vi "test_read-nmea-data2.vi"() -> ()   [LabVIEW 2019] (continued)
A,3,12,06,19,05,17,09,04,02,,,,,1.88,0.95,1.62,1*08\n\t\n15:13:30.30\tF9P\t$GNGSA,A,3,85,70,71,84,,,,,,,,,1.88,0.95,1.62,2*0A\n\t\n15:13:30.32\tF9P\t$GNGSA,A,3,36,19,11,04,09,12,,,,,,,1.88,0.95,1.62,3*08\n\t\n15:13:30.34\tF9P\t$GNGSA,A,3,14,11,33,,,,,,,,,,1.88,0.95,1.62,4*09\n\t\n15:13:30.36\tF9P\t$GPGSV,3,1,09,02,55,320,27,04,17,043,22,05,38,248,31,06,64,050,28,1*65\n\t\n15:13:30.38\tF9P\t$GPGSV,3,2,09,09,44,073,34,12,23,276,36,17,33,154,44,19,52,157,39,1*62\n\t\n15:13:30.40\tF9P\t$GPGSV,3,3,09,25,12,306,24,1*5A\n\t\n15:13:30.42\tF9P\t$GPGSV,3,1,09,02,55,320,,04,17,043,15,05,38,248,15,06,64,050,24,6*69\n\t\n15:13:30.44\tF9P\t$GPGSV,3,2,09,09,44,073,26,12,23,276,22,17,33,154,26,19,52,157,,6*6D\n\t\n15:13:30.46\tF9P\t$GPGSV,3,3,09,25,12,306,,6*5B\n\t\n15:13:30.48\tF9P\t$GLGSV,2,1,08,69,11,031,28,70,70,038,23,71,53,206,28,72,05,210,19,1*7B\n\t\n15:13:30.50\tF9P\t$GLGSV,2,2,08,77,01,325,,84,19,123,21,85,70,070,32,86,37,330,,1*74\n\t\n15:13:30.52\tF9P\t$GLGSV,2,1,08,69,11,031,30,70,70,038,,71,53,206,20,72,05,210,,3*71\n\t\n15:13:30.54\tF9P\t$GLGSV,2,2,08,77,01,325,,84,19,123,27,85,70,070,23,86,37,330,,3*70\n\t\n15:13:30.56\tF9P\t$GAGSV,2,1,08,02,08,297,09,04,66,116,27,09,32,193,27,11,72,359,23,7*7D\n\t\n15:13:30.58\tF9P\t$GAGSV,2,2,08,12,40,103,33,19,26,045,15,25,09,249,17,36,26,308,16,7*7D\n\t\n15:13:30.60\tF9P\t$GAGSV,2,1,08,02,08,297,,04,66,116,,09,32,193,,11,72,359,,2*70\n\t\n15:13:30.62\tF9P\t$GAGSV,2,2,08,12,40,103,,19,26,045,,25,09,249,,36,26,308,,2*7D\n\t\n15:13:30.64\tF9P\t$GBGSV,1,1,04,11,49,132,33,14,87,114,26,28,,,28,33,61,220,27,1*47\n\t\n15:13:30.66\tF9P\t$GBGSV,1,1,03,11,49,132,31,14,87,114,23,33,61,220,,3*40\n\t\n15:13:30.68\tF9P\t$GNGLL,3723.56358,N,12656.98749,E,061332.00,A,A*77\n\t\n15:13:30.70\tF9P\t\t\n15:13:30.72\tF9P\t\t\n15:13:30.74\tF9P\t\t\n15:13:30.76\tF9P\t\t\n15:13:30.78\tF9P\t\t\n15:13:30.80\tF9P\t\t\n15:13:30.82\tF9P\t\t\n15:13:30.84\tF9P\t\t\n15:13:30.86\tF9P\t\t\n15:13:30.88\tF9P\t\t\n15:13:30.90\tF9P\t\t\n15:13:30.92\tF9P\t\t\n15:13:30.94\tF9P\t\t\n15:13:30.96\tF9P\t\t\n15:13:30.98\tF9P\t\t\n15:13:31.00\tF9P\t\t\n15:13:31.02\tF9P\t\t\n15:13:31.04\tF9P\t\t\n15:13:31.06\tF9P\t\t\n15:13:31.08\tF9P\t\t\n15:13:31.10\tF9P\t\t\n15:13:31.12\tF9P\t\t\n15:13:31.14\tF9P\t\t\n15:13:31.16\tF9P\t\t\n15:13:31.18\tF9P\t\t\n15:13:31.20\tF9P\t\t\n15:13:31.22\tF9P\t\t\n15:13:31.24\tF9P\t$GNRMC,061333.00,A,3723.56413,N,12656.98779,E,2.031,10.66,250720,,,A,V*33\n\t\n15:13:31.26\tF9P\t$GNVTG,10.66,T,,M,2.031,N,3.761,K,A*11\n\t\n15:13:31.28\tF9P\t$GNGGA,061333.00,3723.56413,N,12656.98779,E,1,12,0.82,49.3,M,18.5,M,,*73\n\t\n15:13:31.30\tF9P\t$GNGSA,A,3,12,06,19,05,17,09,04,02,,,,,1.52,0.82,1.28,1*07\n\t\n15:13:31.32\tF9P\t$GNGSA,A,3,85,70,71,84,,,,,,,,,1.52,0.82,1.28,2*05\n\t\n15:13:31.34\tF9P\t$GNGSA,A,3,36,19,11,04,09,12,,,,,,,1.52,0.82,1.28,3*07\n\t\n15:13:31.36\tF9P\t$GNGSA,A,3,14,11,33,,,,,,,,,,1.52,0.82,1.28,4*06\n\t\n15:13:31.38\tF9P\t$GPGSV,3,1,09,02,55,320,26,04,17,043,22,05,38,248,25,06,64,050,28,1*61\n\t\n15:13:31.40\tF9P\t$GPGSV,3,2,09,09,44,073,26,12,23,276,33,17,33,154,42,19,52,157,31,1*6A\n\t\n15:13:31.42\tF9P\t$GPGSV,3,3,09,25,12,306,31,1*5E\n\t\n15:13:31.44\tF9P\t$GPGSV,3,1,09,02,55,320,,04,17,043,14,05,38,248,10,06,64,050,24,6*6D\n\t\n15:13:31.46\tF9P\t$GPGSV,3,2,09,09,44,073,26,12,23,276,20,17,33,154,25,19,52,157,,6*6C\n\t\n15:13:31.48\tF9P\t$GPGSV,3,3,09,25,12,306,,6*5B\n\t\n15:13:31.50\tF9P\t$GLGSV,2,1,08,69,11,031,25,70,70,038,22,71,53,206,27,72,05,210,18,1*79\n\t\n15:13:31.52\tF9P\t$GLGSV,2,2,08,77,01,325,,84,19,123,21,85,70,070,32,86,37,330,,1*74\n\t\n15:13:31.54\tF9P\t$GLGSV,2,1,08,69,11,031,26,70,70,038,,71,53,206,19,72,05,210,,3*7C\n\t\n15:13:31.56\tF9P\t$GLGSV,2,2,08,77,01,325,,84,19,123,26,85,70,070,21,86,37,330,,3*73\n\t\n15:13:31.58\tF9P\t$GAGSV,2,1,08,02,08,297,07,04,66,116,27,09,32,193,27,11,72,359,24,7*74\n\t\n15:13:31.60\tF9P\t$GAGSV,2,2,08,12,40,103,29,19,26,045,15,25,09,249,13,36,26,308,16,7*72\n\t\n15:13:31.62\tF9P\t$GAGSV,2,1,08,02,08,297,,04,66,116,,09,32,193,,11,72,359,,2*70\n\t\n15:13:31.64\tF9P\t$GAGSV,2,2,08,12,40,103,,19,26,045,,25,09,249,,36,26,308,,2*7D\n\t\n15:13:31.66\tF9P\t$GBGSV,1,1,04,11,49,132,36,14,87,114,27,28,,,27,33,61,220,27,1*4C\n\t\n15:13:31.68\tF9P\t$GBGSV,1,1,03,11,49,132,30,14,87,114,30,33,61,220,,3*43\n\t\n15:13:31.70\tF9P\t$GNGLL,3723.56413,N,12656.98779,E,061333.00,A,A*7D\n\t\n15:13:31.72\tF9P\t\t\n15:13:31.74\tF9P\t\t\n15:13:31.76\tF9P\t\t\n15:13:31.78\tF9P\t\t\n15:13:31.80\tF9P\t\t\n15:13:31.82\tF9P\t\t\n15:13:31.84\tF9P\t\t\n15:13:31.86\tF9P\t\t\n15:13:31.88\tF9P\t\t\n15:13:31.90\tF9P\t\t\n15:13:31.92\tF9P\t\t\n15:13:31.94\tF9P\t\t\n15:13:31.96\tF9P\t\t\n15:13:31.98\tF9P\t\t\n15:13:32.00\tF9P\t\t\n15:13:32.02\tF9P\t\t\n15:13:32.04\tF9P\t\t\n15:13:32.06\tF9P\t\t\n15:13:32.08\tF9P\t\t\n15:13:32.10\tF9P\t\t\n15:13:32.12\tF9P\t\t\n15:13:32.14\tF9P\t\t\n15:13:32.16\tF9P\t\t\n15:13:32.18\tF9P\t\t\n15:13:32.20\tF9P\t\t\n15:13:32.22\tF9P\t\t\n15:13:32.24\tF9P\t$GNRMC,061334.00,A,3723.56475,N,12656.98800,E,1.899,7.08,250720,,,A,V*02\n\t\n15:13:32.26\tF9P\t$GNVTG,7.08,T,,M,1.899,N,3.517,K,A*25\n\t\n15:13:32.28\tF9P\t$GNGGA,061334.00,3723.56475,N,12656.98800,E,1,12,0.82,49.2,M,18.5,M,,*74\n\t\n15:13:32.30\tF9P\t$GNGSA,A,3,12,06,19,05,17,09,04,02,,,,,1.52,0.82,1.28,1*07\n\t\n15:13:32.32\tF9P\t$GNGSA,A,3,85,70,71,84,,,,,,,,,1.52,0.82,1.28,2*05\n\t\n15:13:32.34\tF9P\t$GNGSA,A,3,36,19,11,04,09,12,,,,,,,1.52,0.82,1.28,3*07\n\t\n15:13:32.36\tF9P\t$GNGSA,A,3,14,11,33,,,,,,,,,,1.52,0.82,1.28,4*06\n\t\n15:13:32.38\tF9P\t$GPGSV,3,1,09,02,55,320,31,04,17,043,22,05,38,248,24,06,64,050,33,1*6C\n\t\n15:13:32.40\tF9P\t$GPGSV,3,2,09,09,44,073,31,12,23,276,37,17,32,154,31,19,52,157,35,1*69\n\t\n15:13:32.42\tF9P\t$GPGSV,3,3,09,25,12,306,24,1*5A\n\t\n15:13:32.44\tF9P\t$GPGSV,3,1,09,02,55,320,,04,17,043,12,05,38,248,,06,64,050,24,6*6A\n\t\n15:13:32.46\tF9P\t$GPGSV,3,2,09,09,44,073,26,12,23,276,20,17,32,154,25,19,52,157,,6*6D\n\t\n15:13:32.48\tF9P\t$GPGSV,3,3,09,25,12,306,,6*5B\n\t\n15:13:32.50\tF9P\t$GLGSV,2,1,08,69,11,031,31,70,70,038,22,71,53,206,28,72,05,210,17,1*7C\n\t\n15:13:32.52\tF9P\t$GLGSV,2,2,08,77,01,325,,84,19,123,19,85,70,070,33,86,37,330,,1*7E\n\t\n15:13:32.54\tF9P\t$GLGSV,2,1,08,69,11,031,26,70,70,038,,71,53,206,18,72,05,210,,3*7D\n\t\n15:13:32.56\tF9P\t$GLGSV,2,2,08,77,01,325,,84,19,123,25,85,70,070,21,86,37,330,,3*70\n\t\n15:13:32.58\tF9P\t$GAGSV,2,1,08,02,08,297,08,04,66,116,31,09,32,193,25,11,72,359,24,7*7E\n\t\n15:13:32.60\tF9P\t$GAGSV,2,2,08,12,40,103,29,19,26,045,16,25,09,249,11,36,26,308,15,7*70\n\t\n15:13:32.62\tF9P\t$GAGSV,2,1,08,02,08,297,,04,66,116,,09,32,193,,11,72,359,,2*70\n\t\n15:13:32.64\tF9P\t$GAGSV,2,2,08,12,40,103,,19,26,045,,25,09,249,,36,26,308,,2*7D\n\t\n15:13:32.66\tF9P\t$GBGSV,1,1,04,11,49,132,33,14,87,114,28,28,,,26,33,61,220,38,1*49\n\t\n15:13:32.68\tF9P\t$GBGSV,1,1,03,11,49,132,,14,87,114,,33,61,220,,3*43\n\t\n15:13:32.70\tF9P\t$GNGLL,3723.56475,N,12656.98800,E,061334.00,A,A*7B\n\t\n15:13:32.72\tF9P\t\t\n15:13:32.74\tF9P\t\t\n15:13:32.76\tF9P\t\t\n15:13:32.78\tF9P\t\t\n15:13:32.80\tF9P\t\t\n15:13:32.82\tF9P\t\t\n15:13:32.84\tF9P\t\t\n15:13:32.86\tF9P\t\t\n15:13:32.88\tF9P\t\t\n15:13:32.90\tF9P\t\t\n15:13:32.92\tF9P\t\t\n15:13:32.94\tF9P\t\t\n15:13:32.96\tF9P\t\t\n15:13:32.98\tF9P\t\t\n15:13:33.00\tF9P\t\t\n15:13:33.02\tF9P\t\t\n15:13:33.04\tF9P\t\t\n15:13:33.06\tF9P\t\t\n15:13:33.08\tF9P\t\t\n15:13:33.10\tF9P\t\t\n15:13:33.12\tF9P\t\t\n15:13:33.14\tF9P\t\t\n15:13:33.16\tF9P\t\t\n15:13:33.18\tF9P\t\t\n15:13:33.20\tF9P\t\t\n15:13:33.22\tF9P\t\t\n15:13:33.24\tF9P\t$GNRMC,061335.00,A,3723.56544,N,12656.98826,E,2.231,5.91,250720,,,A,V*0D\n\t\n15:13:33.26\tF9P\t$GNVTG,5.91,T,,M,2.231,N,4.131,K,A*2B\n\t\n15:13:33.28\tF9P\t$GNGGA,061335.00,3723.56544,N,12656.98826,E,1,12,0.95,49.1,M,18.5,M,,*77\n\t\n15:13:33.30\tF9P\t$GNGSA,A,3,12,06,19,05,17,09,04,02,,,,,1.88,0.95,1.62,1*08\n\t\n15:13:33.32\tF9P\t$GNGSA,A,3,85,70,71,84,,,,,,,,,1.88,0.95,1.62,2*0A\n\t\n15:13:33.34\tF9P\t$GNGSA,A,3,36,19,11,04,09,12,,,,,,,1.88,0.95,1.62,3*08\n\t\n15:13:33.36\tF9P\t$GNGSA,A,3,14,11,33,,,,,,,,,,1.88,0.95,1.62,4*09\n\t\n15:13:33.38\tF9P\t$GPGSV,3,1,09,02,55,320,32,04,17,043,22,05,38,248,25,06,64,050,33,1*6E\n\t\n15:13:33.40\tF9P\t$GPGSV,3,2,09,09,44,073,30,12,23,276,35,17,32,154,39,19,52,157,33,1*64\n\t\n15:13:33.42\tF9P\t$GPGSV,3,3,09,25,12,306,22,1*5C\n\t\n15:13:33.44\tF9P\t$GPGSV,3,1,09,02,55,320,,04,17,043,10,05,38,248,,06,64,050,31,6*6C\n\t\n15:13:33.46\tF9P\t$GPGSV,3,2,09,09,44,073,25,12,23,276,19,17,32,154,25,19,52,157,,6*64\n\t\n15:13:33.48\tF9P\t$GPGSV,3,3,09,25,12,306,,6*5B\n\t\n15:13:33.50\tF9P\t$GLGSV,2,1,08,69,11,031,29,70,70,038,23,71,53,206,35,72,05,210,17,1*78\n\t\n15:13:33.52\tF9P\t$GLGSV,2,2,08,77,01,325,,84,19,123,18,85,70,070,35,86,37,330,,1*79\n\t\n15:13:33.54\tF9P\t$GLGSV,2,1,08,69,11,031,25,70,70,038,,71,53,206,21,72,05,210,,3*74\n\t\n15:13:33.56\tF9P\t$GLGSV,2,2,08,77,01,325,,84,19,123,22,85,70,070,21,86,37,330,,3*77\n\t\n15:13:33.58\tF9P\t$GAGSV,2,1,08,02,08,297,11,04,66,116,24,09,32,193,25,11,72,359,25,7*73\n\t\n15:13:33.60\tF9P\t$GAGSV,2,2,08,12,40,103,28,19,26,045,16,25,09,249,10,36,26,308,14,7*71\n\t\n15:13:33.62\tF9P\t$GAGSV,2,1,08,02,08,297,,04,66,116,,09,32,193,,11,72,359,,2*70\n\t\n15:13:33.64\tF9P\t$GAGSV,2,2,08,12,40,103,,19,26,045,,25,09,249,,36,26,308,,2*7D\n\t\n15:13:33.66\tF9P\t$GBGSV,1,1,04,11,49,132,38,14,87,114,27,28,,,26,33,61,220,35,1*40\n\t\n15:13:33.68\tF9P\t$GBGSV,1,1,03,11,49,132,29,14,87,114,,33,61,220,,3*48\n\t\n15:13:33.70\tF9P\t$GNGLL,3723.56544,N,12656.98826,E,061335.00,A,A*7D\n\t\n15:13:33.72\tF9P\t\t\n15:13:33.74\tF9P\t\t\n15:13:33.76\tF9P\t\t\n15:13:33.78\tF9P\t\t\n15:13:33.80\tF9P\t\t\n15:13:33.82\tF9P\t\t\n15:13:33.84\tF9P\t\t\n15:13:33.86\tF9P\t\t\n15:13:33.88\tF9P\t\t\n15:13:33.90\tF9P\t\t\n15:13:33.92\tF9P\t\t\n15:13:33.94\tF9P\t\t\n15:13:33.96\tF9P\t\t\n15:13:33.98\tF9P\t\t\n15:13:34.00\tF9P\t\t\n15:13:34.02\tF9P\t\t\n15:13:34.04\tF9P\t\t\n15:13:34.06\tF9P\t\t\n15:13:34.08\tF9P\t\t\n15:13:34.10\tF9P\t\t\n15:13:34.12\tF9P\t\t\n15:13:34.14\tF9P\t\t\n15:13:34.16\tF9P\t\t\n15:13:34.18\tF9P\t\t\n15:13:34.20\tF9P\t\t\n15:13:34.22\tF9P\t\t\n15:13:34.24\tF9P\t$GNRMC,061336.00,A,3723.56612,N,12656.98828,E,1.880,2.24,250720,,,A,V*0A\n\t\n15:13:34.26\tF9P\t$GNVTG,2.24,T,,M,1.880,N,3.482,K,A*2B\n\t\n15:13:34.28\tF9P\t$GNGGA,061336.00,3723.56612,N,12656.98828,E,1,12,1.09,48.9,M,18.5,M,,*77\n\t\n15:13:34.30\tF9P\t$GNGSA,A,3,12,06,19,05,17,09,04,02,,,,,2.14,1.09,1.84,1*02\n\t\n15:13:34.32\tF9P\t$GNGSA,A,3,85,70,71,84,,,,,,,,,2.14,1.09,1.84,2*00\n\t\n15:13:34.35\tF9P\t$GNGSA,A,3,36,19,11,04,09,12,,,,,,,2.14,1.09,1.84,3*02\n\t\n15:13:34.37\tF9P\t$GNGSA,A,3,14,11,33,,,,,,,,,,2.14,1.09,1.84,4*03\n\t\n15:13:34.39\tF9P\t$GPGSV,3,1,09,02,55,320,32,04,17,043,20,05,38,248,26,06,64,050,28,1*65\n\t\n15:13:34.41\tF9P\t$GPGSV,3,2,09,09,44,073,32,12,23,276,38,17,32,154,38,19,51,157,29,1*62\n\t\n15:13:34.43\tF9P\t$GPGSV,3,3,09,25,12,306,21,1*5F\n\t\n15:13:34.45\tF9P\t$GPGSV,3,1,09,02,55,320,,04,17,043,11,05,38,248,,06,64,050,25,6*68\n\t\n15:13:34.47\tF9P\t$GPGSV,3,2,09,09,44,073,25,12,23,276,19,17,32,154,24,19,51,157,,6*66\n\t\n15:13:34.49\tF9P\t$GPGSV,3,3,09,25,12,306,,6*5B\n\t\n15:13:34.51\tF9P\t$GLGSV,2,1,08,69,11,031,28,70,70,038,24,71,53,206,33,72,05,210,18,1*77\n\t\n15:13:34.53\tF9P\t$GLGSV,2,2,08,77,01,325,,84,19,123,19,85,70,070,38,86,37,330,,1*75\n\t\n15:13:34.55\tF9P\t$GLGSV,2,1,08,69,11,031,23,70,70,038,,71,53,206,25,72,05,210,,3*76\n\t\n15:13:34.57\tF9P\t$GLGSV,2,2,08,77,01,325,,84,19,123,21,85,70,070,21,86,37,330,,3*74\n\t\n15:13:34.59\tF9P\t$GAGSV,2,1,08,02,08,297,07,04,66,116,26,09,32,193,34,11,72,359,26,7*75\n\t\n15:13:34.61\tF9P\t$GAGSV,2,2,08,12,40,103,28,19,26,045,17,25,09,249,10,36,26,308,14,7*70\n\t\n15:13:34.63\tF9P\t$GAGSV,2,1,08,02,08,297,,04,66,116,,09,32,193,,11,72,359,,2*70\n\t\n15:13:34.65\tF9P\t$GAGSV,2,2,08,12,40,103,,19,26,045,,25,09,249,,36,26,308,,2*7D\n\t\n15:13:34.67\tF9P\t$GBGSV,1,1,04,11,49,132,30,14,87,114,27,28,,,27,33,61,220,33,1*4F\n\t\n15:13:34.69\tF9P\t$GBGSV,1,1,03,11,49,132,,14,87,114,,33,61,220,,3*43\n\t\n15:13:34.71\tF9P\t$GNGLL,3723.56612,N,12656.98828,E,061336.00,A,A*70\n\t\n15:13:34.73\tF9P\t\t\n15:13:34.75\tF9P\t\t\n15:13:34.77\tF9P\t\t\n15:13:34.79\tF9P\t\t\n15:13:34.81\tF9P\t\t\n15:13:34.83\tF9P\t\t\n15:13:34.85\tF9P\t\t\n15:13:34.87\tF9P\t\t\n15:13:34.89\tF9P\t\t\n15:13:34.91\tF9P\t\t\n15:13:34.93\tF9P\t\t\n15:13:34.95\tF9P\t\t\n15:13:34.97\tF9P\t\t\n15:13:34.99\tF9P\t\t\n15:13:35.01\tF9P\t\t\n15:13:35.03\tF9P\t\t\n15:13:35.05\tF9P\t\t\n15:13:35.07\tF9P\t\t\n15:13:35.09\tF9P\t\t\n15:13:35.11\tF9P\t\t\n15:13:35.13\tF9P\t\t\n15:13:35.15\tF9P\t\t\n15:13:35.17\tF9P\t\t\n15:13:35.19\tF9P\t\t\n15:13:35.21\tF9P\t\t\n15:13:35.23\tF9P\t$GNRMC,061337.00,A,3723.56656,N,12656.98836,E,1.514,358.52,250720,,,A,V*09\n\t\n15:13:35.25\tF9P\t$GNVTG,358.52,T,,M,1.514,N,2.804,K,A*25\n\t\n15:13:35.27\tF9P\t$GNGGA,061337.00,3723.56656,N,12656.98836,E,1,12,1.09,49.1,M,18.5,M,,*70\n\t\n15:13:35.29\tF9P\t$GNGSA,A,3,12,06,19,05,17,09,04,02,,,,,2.14,1.09,1.84,1*02\n\t\n15:13:35.31\tF9P\t$GNGSA,A,3,85,70,71,84,,,,,,,,,2.14,1.09,1.84,2*00\n\t\n15:13:35.33\tF9P\t$GNGSA,A,3,36,19,11,04,09,12,,,,,,,2.14,1.09,1.84,3*02\n\t\n15:13:35.35\tF9P\t$GNGSA,A,3,14,11,33,,,,,,,,,,2.14,1.09,1.84,4*03\n\t\n15:13:35.37\tF9P\t$GPGSV,3,1,09,02,55,320,27,04,17,043,19,05,38,248,26,06,64,050,34,1*66\n\t\n15:13:35.39\tF9P\t$GPGSV,3,2,09,09,44,073,27,12,23,276,31,17,32,154,31,19,51,157,32,1*6C\n\t\n15:13:35.41\tF9P\t$GPGSV,3,3,09,25,12,306,22,1*5C\n\t\n15:13:35.43\tF9P\t$GPGSV,3,1,09,02,55,320,,04,17,043,10,05,38,248,,06,64,050,26,6*6A\n\t\n15:13:35.45\tF9P\t$GPGSV,3,2,09,09,44,073,27,12,23,276,18,17,32,154,25,19,51,157,,6*64\n\t\n15:13:35.47\tF9P\t$GPGSV,3,3,09,25,12,306,,6*5B\n\t\n15:13:35.49\tF9P\t$GLGSV,2,1,08,69,11,031,28,70,70,038,25,71,53,206,31,72,05,210,18,1*74\n\t\n15:13:35.51\tF9P\t$GLGSV,2,2,08,77,01,325,,84,19,123,19,85,70,070,32,86,37,330,,1*7F\n\t\n15:13:35.53\tF9P\t$GLGSV,2,1,08,69,11,031,22,70,70,038,,71,53,206,25,72,05,210,,3*77\n\t\n15:13:35.55\tF9P\t$GLGSV,2,2,08,77,01,325,,84,19,123,21,85,70,070,24,86,37,330,,3*71\n\t\n15:13:35.57\tF9P\t$GAGSV,2,1,08,02,08,297,07,04,66,116,32,09,32,193,31,11,72,359,24,7*77\n\t\n15:13:35.59\tF9P\t$GAGSV,2,2,08,12,40,103,28,19,26,045,17,25,09,249,09,36,26,308,13,7*7F\n\t\n15:13:35.61\tF9P\t$GAGSV,2,1,08,02,08,297,,04,66,116,,09,32,193,,11,72,359,,2*70\n\t\n15:13:35.63\tF9P\t$GAGSV,2,2,08,12,40,103,,19,26,045,,25,09,249,,36,26,308,,2*7D\n\t\n15:13:35.65\tF9P\t$GBGSV,1,1,04,11,49,132,33,14,87,114,32,28,,,27,33,61,220,35,1*4E\n\t\n15:13:35.67\tF9P\t$GBGSV,1,1,03,11,49,132,,14,87,114,31,33,61,220,,3*41\n\t\n15:13:35.69\tF9P\t$GNGLL,3723.56656,N,12656.98836,E,061337.00,A,A*7E\n\t\n15:13:35.71\tF9P\t\t\n15:13:35.73\tF9P\t\t\n15:13:35.75\tF9P\t\t\n15:13:35.77\tF9P\t\t\n15:13:35.79\tF9P\t\t\n15:13:35.81\tF9P\t\t\n15:13:35.83\tF9P\t\t\n15:13:35.85\tF9P\t\t\n15:13:35.87\tF9P\t\t\n15:13:35.89\tF9P\t\t\n15:13:35.91\tF9P\t\t\n15:13:35.93\tF9P\t\t\n15:13:35.95\tF9P\t\t\n15:13:35.97\tF9P\t\t\n15:13:35.99\tF9P\t\t\n15:13:36.01\tF9P\t\t\n15:13:36.03\tF9P\t\t\n15:13:36.05\tF9P\t\t\n15:13:36.07\tF9P\t\t\n15:13:36.09\tF9P\t\t\n15:13:36.11\tF9P\t\t\n15:13:36.13\tF9P\t\t\n15:13:36.15\tF9P\t\t\n15:13:36.17\tF9P\t\t\n15:13:36.19\tF9P\t\t\n15:13:36.21\tF9P\t\t\n15:13:36.23\tF9P\t$GNRMC,061338.00,A,3723.56740,N,12656.98792,E,2.771,332.85,250720,,,A,V*05\n\t\n15:13:36.25\tF9P\t$GNVTG,332.85,T,,M,2.771,N,5.132,K,A*2A\n\t\n15:13:36.27\tF9P\t$GNGGA,061338.00,3723.56740,N,12656.98792,E,1,12,0.82,47.5,M,18.5,M,,*70\n\t\n15:13:36.29\tF9P\t$GNGSA,A,3,12,06,19,05,17,09,04,02,,,,,1.52,0.82,1.28,1*07\n\t\n15:13:36.31\tF9P\t$GNGSA,A,3,85,70,71,84,,,,,,,,,1.52,0.82,1.28,2*05\n\t\n15:13:36.33\tF9P\t$GNGSA,A,3,36,19,11,04,09,12,,,,,,,1.52,0.82,1.28,3*07\n\t\n15:13:36.35\tF9P\t$GNGSA,A,3,14,11,33,,,,,,,,,,1.52,0.82,1.28,4*06\n\t\n15:13:36.37\tF9P\t$GPGSV,3,1,09,02,55,320,34,04,17,043,18,05,38,248,26,06,64,050,30,1*61\n\t\n15:13:36.39\tF9P\t$GPGSV,3,2,09,09,44,073,30,12,23,276,35,17,32,154,36,19,51,157,32,1*69\n\t\n15:13:36.41\tF9P\t$GPGSV,3,3,09,25,12,306,21,1*5F\n\t\n15:13:36.43\tF9P\t$GPGSV,3,1,09,02,55,320,,04,17,043,,05,38,248,,06,64,050,26,6*6B\n\t\n15:13:36.45\tF9P\t$GPGSV,3,2,09,09,44,073,27,12,23,276,21,17,32,154,24,19,51,157,,6*6F\n\t\n15:13:36.47\tF9P\t$GPGSV,3,3,09,25,12,306,,6*5B\n\t\n15:13:36.49\tF9P\t$GLGSV,2,1,08,69,11,031,27,70,70,038,24,71,53,206,30,72,05,210,16,1*75\n\t\n15:13:36.51\tF9P\t$GLGSV,2,2,08,77,01,325,,84,19,123,17,85,70,070,27,86,37,330,,1*75\n\t\n15:13:36.53\tF9P\t$GLGSV,2,1,08,69,11,031,21,70,70,038,,71,53,206,24,72,05,210,,3*75\n\t\n15:13:36.55\tF9P\t$GLGSV,2,2,08,77,01,325,,84,19,123,22,85,70,070,26,86,37,330,,3*70\n\t\n15:13:36.57\tF9P\t$GAGSV,2,1,08,02,08,297,09,04,66,116,32,09,32,193,30,11,72,359,23,7*7F\n\t\n15:13:36.59\tF9P\t$GAGSV,2,2,08,12,40,103,30,19,26,045,16,25,09,249,,36,26,308,13,7*7E\n\t\n15:13:36.61\tF9P\t$GAGSV,2,1,08,02,08,297,,04,66,116,,09,32,193,,11,72,359,,2*70\n\t\n15:13:36.63\tF9P\t$GAGSV,2,2,08,12,40,103,,19,26,045,,25,09,249,,36,26,308,,2*7D\n\t\n15:13:36.65\tF9P\t$GBGSV,1,1,04,11,49,132,33,14,87,114,28,28,,,32,33,61,220,29,1*4C\n\t\n15:13:36.67\tF9P\t$GBGSV,1,1,03,11,49,132,,14,87,114,,33,61,220,,3*43\n\t\n15:13:36.69\tF9P\t$GNGLL,3723.56740,N,12656.98792,E,061338.00,A,A*76\n\t\n15:13:36.71\tF9P\t\t\n15:13:36.73\tF9P\t\t\n15:13:36.75\tF9P\t\t\n15:13:36.77\tF9P\t\t\n15:13:36.79\tF9P\t\t\n15:13:36.81\tF9P\t\t\n15:13:36.83\tF9P\t\t\n15:13:36.85\tF9P\t\t\n15:13:36.87\tF9P\t\t\n15:13:36.89\tF9P\t\t\n15:13:36.91\tF9P\t\t\n15:13:36.93\tF9P\t\t\n15:13:36.95\tF9P\t\t\n15:13:36.97\tF9P\t\t\n15:13:36.99\tF9P\t\t\n15:13:37.01\tF9P\t\t\n15:13:37.03\tF9P\t\t\n15:13:37.05\tF9P\t\t\n15:13:37.07\tF9P\t\t\n15:13:37.09\tF9P\t\t\n15:13:37.11\tF9P\t\t\n15:13:37.13\tF9P\t\t\n15:13:37.15\tF9P\t\t\n15:13:37.17\tF9P\t\t\n15:13:37.19\tF9P\t\t\n15:13:37.21\tF9P\t\t\n15:13:37.23\tF9P\t$GNRMC,061339.00,A,3723.56803,N,12656.98784,E,2.447,331.86,250720,,,A,V*0D\n\t\n15:13:37.25\tF9P\t$GNVTG,331.86,T,,M,2.447,N,4.531,K,A*2A\n\t\n15:13:37.27\tF9P\t$GNGGA,061339.00,3723.56803,N,12656.98784,E,1,12,0.82,47.9,M,18.5,M,,*72\n\t\n15:13:37.29\tF9P\t$GNGSA,A,3,12,06,19,05,17,09,04,02,,,,,1.52,0.82,1.28,1*07\n\t\n15:13:37.31\tF9P\t$GNGSA,A,3,85,70,71,84,,,,,,,,,1.52,0.82,1.28,2*05\n\t\n15:13:37.33\tF9P\t$GNGSA,A,3,36,19,11,04,09,12,,,,,,,1.52,0.82,1.28,3*07\n\t\n15:13:37.35\tF9P\t$GNGSA,A,3,14,11,33,,,,,,,,,,1.52,0.82,1.28,4*06\n\t\n15:13:37.37\tF9P\t$GPGSV,3,1,09,02,55,320,29,04,17,043,18,05,38,248,26,06,64,050,30,1*6D\n\t\n15:13:37.39\tF9P\t$GPGSV,3,2,09,09,44,073,36,12,23,276,33,17,32,154,32,19,51,157,29,1*67\n\t\n15:13:37.41\tF9P\t$GPGSV,3,3,09,25,12,306,22,1*5C\n\t\n15:13:37.43\tF9P\t$GPGSV,3,1,09,02,55,320,,04,17,043,,05,38,248,,06,64,050,25,6*68\n\t\n15:13:37.45\tF9P\t$GPGSV,3,2,09,09,44,073,28,12,23,276,21,17,32,154,24,19,51,157,,6*60\n\t\n15:13:37.47\tF9P\t$GPGSV,3,3,09,25,12,306,,6*5B\n\t\n15:13:37.49\tF9P\t$GLGSV,2,1,08,69,11,031,19,70,70,038,23,71,53,206,33,72,05,210,17,1*7D\n\t\n15:13:37.51\tF9P\t$GLGSV,2,2,08,77,01,325,,84,19,123,18,85,70,070,32,86,37,330,,1*7E\n\t\n15:13:37.53\tF9P\t$GLGSV,2,1,08,69,11,031,21,70,70,038,,71,53,206,30,72,05,210,,3*70\n\t\n15:13:37.55\tF9P\t$GLGSV,2,2,08,77,01,325,,84,19,123,22,85,70,070,24,86,37,330,,3*72\n\t\n15:13:37.57\tF9P\t$GAGSV,2,1,08,02,08,297,09,04,66,116,33,09,32,193,35,11,72,359,22,7*7A\n\t\n15:13:37.59\tF9P\t$GAGSV,2,2,08,12,40,103,34,19,26,045,16,25,09,249,,36,26,308,12,7*7B\n\t\n15:13:37.61\tF9P\t$GAGSV,2,1,08,02,08,297,,04,66,116,,09,32,193,,11,72,359,,2*70\n\t\n15:13:37.63\tF9P\t$GAGSV,2,2,08,12,40,103,,19,26,045,,25,09,249,,36,26,308,,2*7D\n\t\n15:13:37.65\tF9P\t$GBGSV,1,1,04,11,49,132,36,14,87,114,27,28,,,28,33,61,220,29,1*4D\n\t\n15:13:37.67\tF9P\t$GBGSV,1,1,03,11,49,132,,14,87,114,,33,61,220,,3*43\n\t\n15:13:37.69\tF9P\t$GNGLL,3723.56803,N,12656.98784,E,061339.00,A,A*78\n\t\n15:13:37.71\tF9P\t\t\n15:13:37.73\tF9P\t\t\n15:13:37.75\tF9P\t\t\n15:13:37.77\tF9P\t\t\n15:13:37.79\tF9P\t\t\n15:13:37.81\tF9P\t\t\n15:13:37.83\tF9P\t\t\n15:13:37.85\tF9P\t\t\n15:13:37.87\tF9P\t\t\n15:13:37.89\tF9P\t\t\n15:13:37.91\tF9P\t\t\n15:13:37.93\tF9P\t
